vi "LVClass_SlopesPostProcessList AddProcessorTabWithHandle.vi"(0 "SlopesPostProcessorList in":refnum<class "SlopesPostProcessorList.lvclass">, 7 "Processing list in":T1[](array[typedef]), 11 "error in (no error)":errorcluster) -> (4 "SlopesPostProcessorList out":refnum<class "SlopesPostProcessorList.lvclass">, 15 "error out":errorcluster)   [LabVIEW 2020, in "SlopesPostProcessorList.lvclass"]
uses:
  SlopesPostProcessorList.lvclass
  Controls/SlopesPostProcessorList - ONE - with handle.ctl
  HasoSlopes/HasoSlopes.lvclass
  Pupil/Pupil.lvclass
  Controls/SlopesPostProcessorList - Filter.ctl
  Controls/SlopesPostProcessorList - Add lens.ctl
  Controls/SlopesPostProcessorList - Double passage.ctl
  Controls/SlopesPostProcessorList - Modulator.ctl
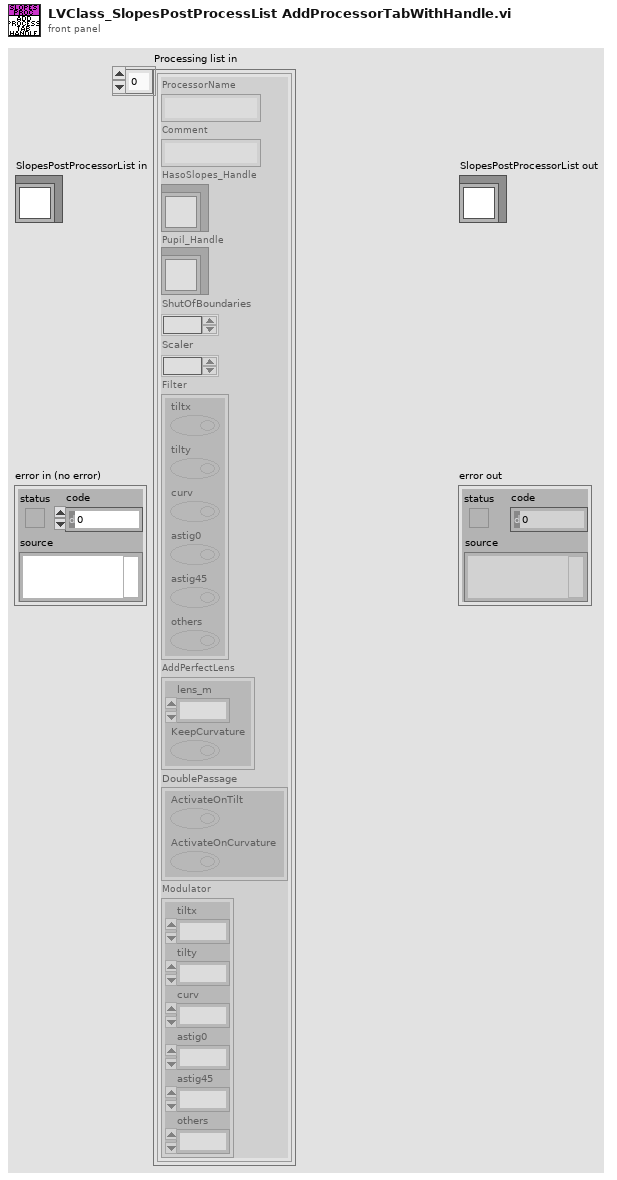
[diagram p1: front panel]
types:
  T1 = typedef "SlopesPostProcessorList - ONE - with handle.ctl" = cluster{"ProcessorName":string, "Comment":string, "HasoSlopes_Handle":refnum<class "HasoSlopes.lvclass">, "Pupil_Handle":refnum<class "Pupil.lvclass">, "ShutOfBoundaries":u16, "Scaler":sgl, "Filter":T2, "AddPerfectLens":T3, "DoublePassage":T4, "Modulator":T5}
  T2 = typedef "SlopesPostProcessorList - Filter.ctl" = cluster{"tiltx":bool, "tilty":bool, "curv":bool, "astig0":bool, "astig45":bool, "others":bool}
  T3 = typedef "SlopesPostProcessorList - Add lens.ctl" = cluster{"lens_m":sgl, "KeepCurvature":bool}
  T4 = typedef "SlopesPostProcessorList - Double passage.ctl" = cluster{"ActivateOnTilt":bool, "ActivateOnCurvature":bool}
  T5 = typedef "SlopesPostProcessorList - Modulator.ctl" = cluster{"tiltx":sgl, "tilty":sgl, "curv":sgl, "astig0":sgl, "astig45":sgl, "others":sgl}
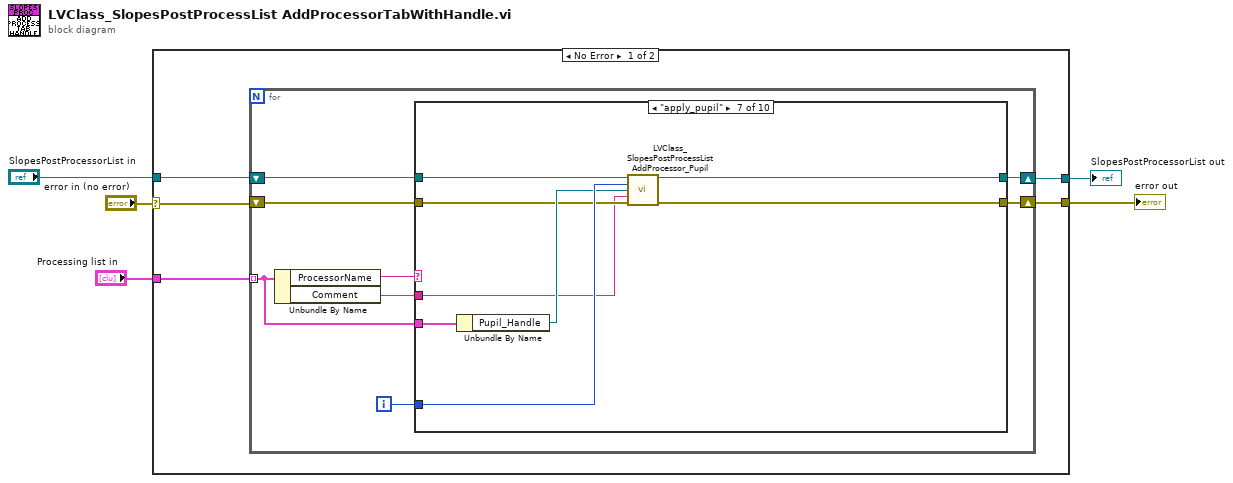
[diagram p0: block diagram]
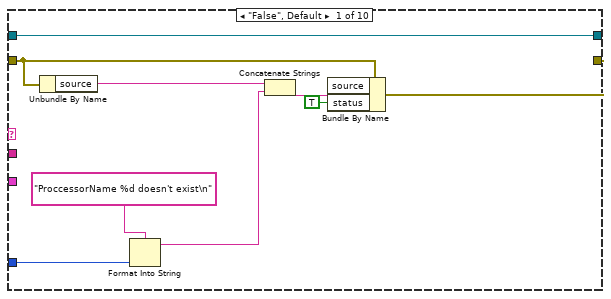
[diagram p2: hidden frame]
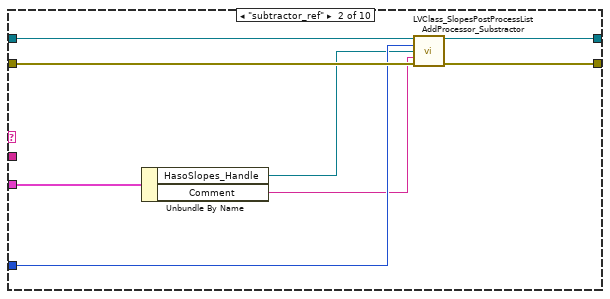
[diagram p3: hidden frame]
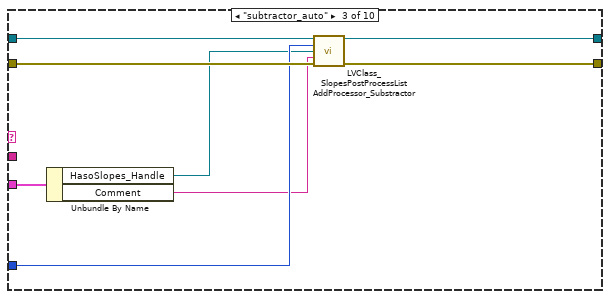
[diagram p4: hidden frame]
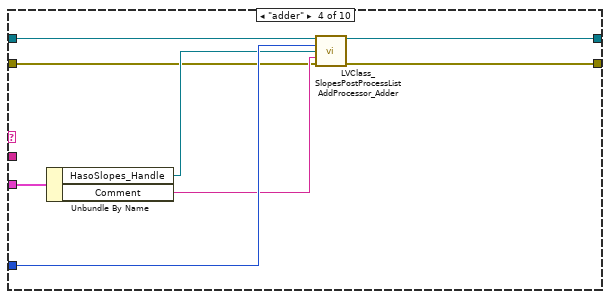
[diagram p5: hidden frame]
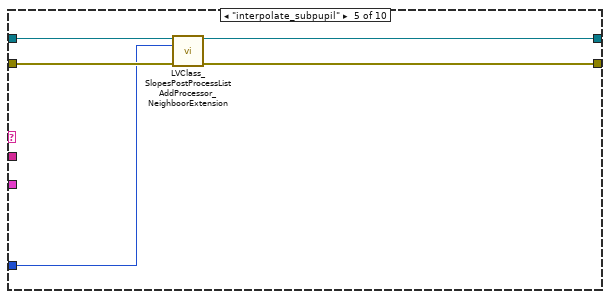
[diagram p6: hidden frame]
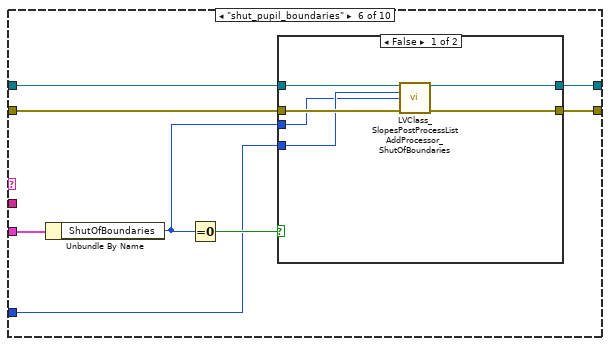
[diagram p7: hidden frame]
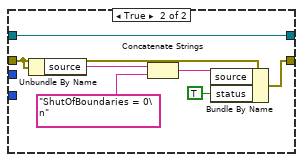
[diagram p8: hidden frame]
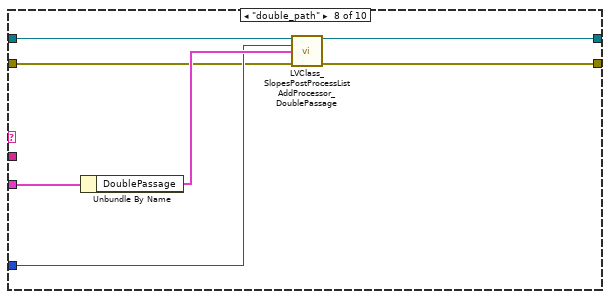
[diagram p9: hidden frame]
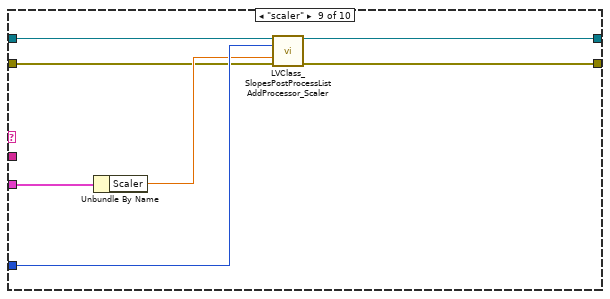
[diagram p10: hidden frame]
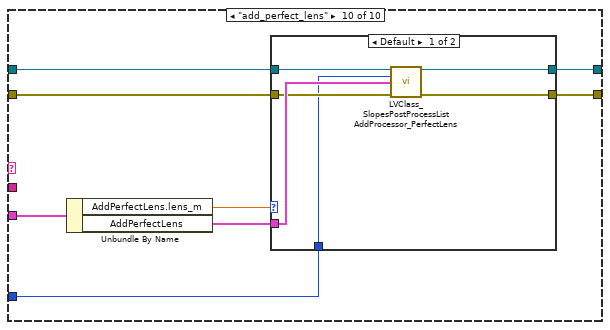
[diagram p11: hidden frame]
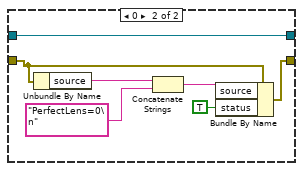
[diagram p12: hidden frame]
diagram:
  n1 = case shown="No Error" "error in (no error)" {
    selector: "error in (no error)" -> [w10 w122]
    tunnel: [w6 w122] -> w4
    tunnel: [w7 w121] -> w5
    tunnel: "SlopesPostProcessorList in" -> [w8 w121]
    tunnel: "Processing list in" -> [w9 _]
    frame No Error {
      n2 = for {
        tunnel: w9 -> [w17] mode=indexing
        shift-right: [w15] -> w6
        shift-left: w10 -> [w16]
        shift-right: [w12] -> w7
        shift-left: w8 -> [w13]
        i -> [w14]
        n3 = Unbundle By Name(w17) -> ("ProcessorName"=w18:string, "Comment"=w11:string)
        n4 = case shown="\"apply_pupil\"" w18 {
          tunnel: w17 -> [_ w35 w43 w51 _ w64 w85 w92 w99 w107]
          tunnel: w16 -> [w27 w34 w42 w45 w54 w62 w79 w87 w94 w105]
          tunnel: [w26 w33 w41 w44 w53 w61 w84 w86 w93 w106] -> w15
          tunnel: w14 -> [w22 w30 w38 w48 w52 w58 w82 w90 w96 w100]
          tunnel: w13 -> [w19 w32 w40 w50 w56 w60 w81 w89 w98 w102]
          tunnel: [w19 w31 w39 w49 w55 w59 w83 w88 w97 w101] -> w12
          tunnel: w11 -> [_ _ _ _ _ _ w78 _ _ _]
          frame "False", Default {
            n5 = Unbundle By Name(w27) -> ("source"=w24:string)
            n6 = Format Into String(format string="ProccessorName %d doesn't exist\n" ("source"), w22) -> (resulting string=w21:string)  [unwired: 2 in, 1 out]
            n7 = Concatenate Strings(w24, w21) -> (w23:string)
            n8 = Bundle By Name(cluster=w27, "source"=w23, "status"=TRUE) -> (w26:errorcluster)
          }
          frame "subtractor_ref" {
            n9 = Unbundle By Name(w35) -> ("HasoSlopes_Handle"=w29:refnum<class "HasoSlopes.lvclass">, "Comment"=w28:string)
            n10 = call "LVClass_SlopesPostProcessList AddProcessor_Substractor.vi"("SlopesPostProcessorList in"=w32, "Position"=w30, "HasoSlopes.lvclass"=w29, "Comment"=w28, "error in (no error)"=w34) -> ("SlopesPostProcessorList out"=w31:refnum<class "SlopesPostProcessorList.lvclass">, "error out"=w33:errorcluster)  [unwired: 9 in]
          }
          frame "subtractor_auto" {
            n11 = Unbundle By Name(w43) -> ("HasoSlopes_Handle"=w37:refnum<class "HasoSlopes.lvclass">, "Comment"=w36:string)
            n12 = call "LVClass_SlopesPostProcessList AddProcessor_Substractor.vi"("SlopesPostProcessorList in"=w40, "Position"=w38, "HasoSlopes.lvclass"=w37, "Comment"=w36, "error in (no error)"=w42) -> ("SlopesPostProcessorList out"=w39:refnum<class "SlopesPostProcessorList.lvclass">, "error out"=w41:errorcluster)  [unwired: 9 in]
          }
          frame "adder" {
            n13 = Unbundle By Name(w51) -> ("HasoSlopes_Handle"=w46:refnum<class "HasoSlopes.lvclass">, "Comment"=w47:string)
            n14 = call "LVClass_SlopesPostProcessList AddProcessor_Adder.vi"("SlopesPostProcessorList in"=w50, "Position"=w48, "HasoSlopes.lvclass"=w46, "Comment"=w47, "error in (no error)"=w45) -> ("SlopesPostProcessorList out"=w49:refnum<class "SlopesPostProcessorList.lvclass">, "error out"=w44:errorcluster)  [unwired: 9 in]
          }
          frame "interpolate_subpupil" {
            n15 = call "LVClass_SlopesPostProcessList AddProcessor_NeighboorExtension.vi"("SlopesPostProcessorList in"=w56, "Position"=w52, "error in (no error)"=w54) -> ("SlopesPostProcessorList out"=w55:refnum<class "SlopesPostProcessorList.lvclass">, "error out"=w53:errorcluster)  [unwired: 11 in]
          }
          frame "shut_pupil_boundaries" {
            n16 = Unbundle By Name(w64) -> ("ShutOfBoundaries"=w57:u16)
            n17 = Equal To 0?(x=w57) -> (x = 0?=w63:bool)
            n18 = case shown="False" w63 {
              tunnel: w62 -> [w69 w72]
              tunnel: [w68 w73] -> w61
              tunnel: w60 -> [w70 w71]
              tunnel: [w67 w71] -> w59
              tunnel: w58 -> [w66 _]
              tunnel: w57 -> [w65 _]
              frame False {
                n19 = call "LVClass_SlopesPostProcessList AddProcessor_ShutOfBoundaries.vi"("SlopesPostProcessorList in"=w70, "Position"=w66, "ShutOfBoundaries"=w65, "error in (no error)"=w69) -> ("SlopesPostProcessorList out"=w67:refnum<class "SlopesPostProcessorList.lvclass">, "error out"=w68:errorcluster)  [unwired: 10 in]
              }
              frame True {
                n20 = Unbundle By Name(w72) -> ("source"=w76:string)
                n21 = Concatenate Strings(w76, "ShutOfBoundaries = 0\n" ("source")) -> (w75:string)
                n22 = Bundle By Name(cluster=w72, "source"=w75, "status"=TRUE) -> (w73:errorcluster)
              }
            }
          }
          frame "apply_pupil" {
            n23 = Unbundle By Name(w85) -> ("Pupil_Handle"=w80:refnum<class "Pupil.lvclass">)
            n24 = call "LVClass_SlopesPostProcessList AddProcessor_Pupil.vi"("SlopesPostProcessorList in"=w81, "Position"=w82, "Pupil.lvclass"=w80, "Comment"=w78, "error in (no error)"=w79) -> ("SlopesPostProcessorList out"=w83:refnum<class "SlopesPostProcessorList.lvclass">, "error out"=w84:errorcluster)  [unwired: 9 in]
          }
          frame "double_path" {
            n25 = Unbundle By Name(w92) -> ("DoublePassage"=w91:T4)
            n26 = call "LVClass_SlopesPostProcessList AddProcessor_DoublePassage.vi"("SlopesPostProcessorList in"=w89, "Position"=w90, "doublePath"=w91, "error in (no error)"=w87) -> ("SlopesPostProcessorList out"=w88:refnum<class "SlopesPostProcessorList.lvclass">, "error out"=w86:errorcluster)  [unwired: 10 in]
          }
          frame "scaler" {
            n27 = Unbundle By Name(w99) -> ("Scaler"=w95:sgl)
            n28 = call "LVClass_SlopesPostProcessList AddProcessor_Scaler.vi"("SlopesPostProcessorList in"=w98, "Position"=w96, "scaler"=w95, "error in (no error)"=w94) -> ("SlopesPostProcessorList out"=w97:refnum<class "SlopesPostProcessorList.lvclass">, "error out"=w93:errorcluster)  [unwired: 10 in]
          }
          frame "add_perfect_lens" {
            n29 = Unbundle By Name(w107) -> ("AddPerfectLens.lens_m"=w104:sgl, "AddPerfectLens"=w103:T3)
            n30 = case shown="Default" w104 {
              tunnel: w105 -> [w109 w117]
              tunnel: [w110 w116] -> w106
              tunnel: w103 -> [w113 _]
              tunnel: w102 -> [w112 w114]
              tunnel: [w111 w114] -> w101
              tunnel: w100 -> [w108 _]
              frame Default {
                n31 = call "LVClass_SlopesPostProcessList AddProcessor_PerfectLens.vi"("SlopesPostProcessorList in"=w112, "Position"=w108, "Perfect lens"=w113, "error in (no error)"=w109) -> ("SlopesPostProcessorList out"=w111:refnum<class "SlopesPostProcessorList.lvclass">, "error out"=w110:errorcluster)  [unwired: 10 in]
              }
              frame 0 {
                n32 = Unbundle By Name(w117) -> ("source"=w119:string)
                n33 = Concatenate Strings(w119, "PerfectLens=0\n" ("source")) -> (w118:string)
                n34 = Bundle By Name(cluster=w117, "source"=w118, "status"=TRUE) -> (w116:errorcluster)
              }
            }
          }
        }
      }
    }
    frame Error {
    }
  }
  "error out" <- w4
  "SlopesPostProcessorList out" <- w5
